vi "PAM Hex String to 16 Bit Number.vi"(10 "Signed?":bool, 11 "Hex String":string="ï;") -> (2 "Signed 16 Bit":i16, 3 "Unsigned 16 Bit":u16)   [LabVIEW 2020]
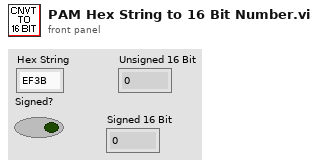
[diagram p1: front panel]
types:
  T1 = enum16{"big-endian, network order", "native, host order", "little-endian"}
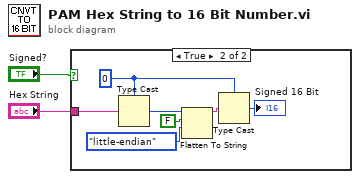
[diagram p0: block diagram]
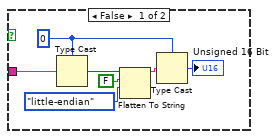
[diagram p2: hidden frame]
diagram:
  n1 = case shown="True" "Signed?" {
    tunnel: "Hex String" -> [w4 w10]
    frame False {
      w5 = u16 0
      n2 = Type Cast(type=w5, x=w4) -> (*(type *) &x=w9:u16)
      n3 = Flatten To String(anything=w9, prepend array or string size? (T)=FALSE, byte order (0:big-endian, network order)=T1."little-endian") -> (data string=w6:string)  [unwired: 1 in, 2 out]
      n4 = Type Cast(type=w5, x=w6) -> (*(type *) &x=→"Unsigned 16 Bit":u16)
    }
    frame True {
      w12 = i16 0
      n5 = Type Cast(type=w12, x=w10) -> (*(type *) &x=w16:i16)
      n6 = Flatten To String(anything=w16, prepend array or string size? (T)=FALSE, byte order (0:big-endian, network order)=T1."little-endian") -> (data string=w13:string)  [unwired: 1 in, 2 out]
      n7 = Type Cast(type=w12, x=w13) -> (*(type *) &x=→"Signed 16 Bit":i16)
    }
  }
